vi "Kinesis_XY-AndreTec-Kelly.vi"() -> ()   [LabVIEW 2014]
panel:
  out "Progresso 2":i32=5
  out "Y 4":sgl=0.9991
  out "X 4":sgl=1.0
  out "Y 3":sgl=0.8991
  out "X 3":sgl=0.0001 format="%#_4g"
  out "Tempo de 1 linha 2":u32=9994
  out "Y 2":sgl=0.9991
  out "Y 1":sgl=0.8991
  out "Tempo de 1 linha":u32=10015
  out "X 2":sgl
  out "X 1":sgl=0.999 format="%#_4g"
  in  "Cronometro":bool
  out "millisecond":sgl=332.872
  in  "Aceleração":dbl=1.0
  in  "d (mm)":sgl=0.1
  in  "L (mm)":sgl=1.0
  in  "Iniciar":bool
  out "Progresso":i32=5
  in  "Numero deCiclos":i32=5
  in  "Velocidade":sgl=0.05
  out "Motor Y\nLigado":bool=TRUE
  out "Motor X \nLigado":bool=TRUE
  # "(mm/s)"
  # "(mm/s.s)"
  # "FOCO"
  # "Não Mover"
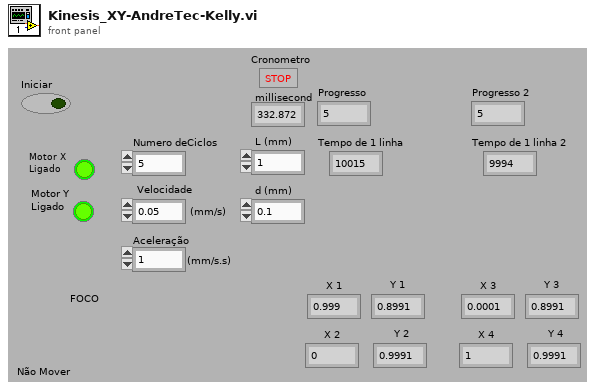
[diagram p1: front panel]
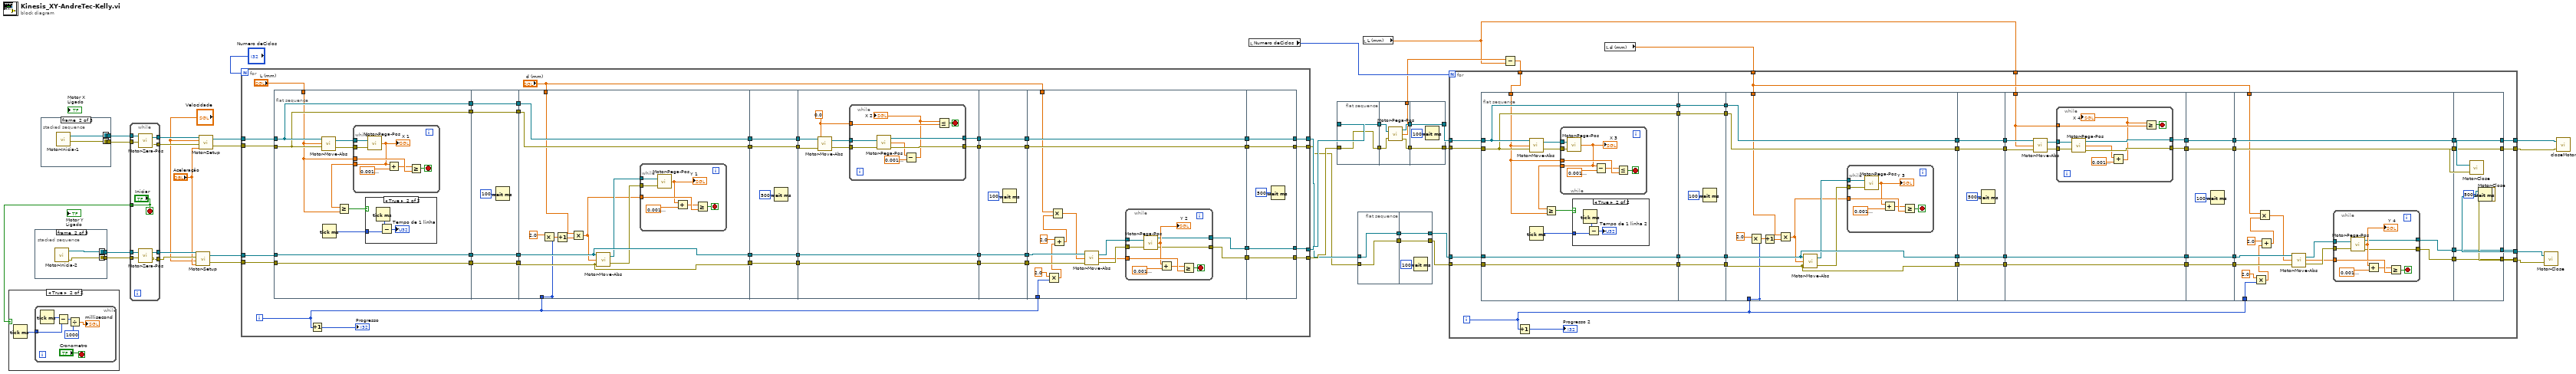
[diagram p0: block diagram]
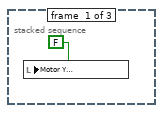
[diagram p5: hidden frame]
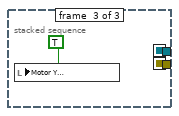
[diagram p6: hidden frame]
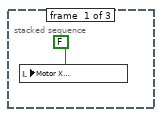
[diagram p7: hidden frame]
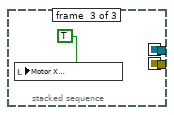
[diagram p8: hidden frame]
diagram:
  n1 = stacked-sequence {
    seq-local: [_ w42 _] -> [_ _ w45]
    seq-local: [_ w41 _] -> [_ _ w44]
    tunnel: [_ _ w45] -> w37
    tunnel: [_ _ w44] -> w36
    frame #0 {
      n2 = local write "Motor Y\nLigado"(FALSE ("Motor3\nLigado")) -> ()
    }
    frame #1 {
      n3 = call "Motor-Inicia-2.vi"() -> ("MG17Motor 2"=w42:refnum<k7>, "error out"=w41:errorcluster)  [unwired: 2 in]
    }
    frame #2 {
      n4 = local write "Motor Y\nLigado"(TRUE ("Motor3\nLigado")) -> ()
    }
  }
  n5 = stacked-sequence {
    seq-local: [_ w48 _] -> [_ _ w51]
    seq-local: [_ w47 _] -> [_ _ w50]
    tunnel: [_ _ w51] -> w39
    tunnel: [_ _ w50] -> w38
    frame #0 {
      n6 = local write "Motor X \nLigado"(FALSE ("x = y?")) -> ()
    }
    frame #1 {
      n7 = call "Motor-Inicia-1.vi"() -> ("MG17Motor 2"=w48:refnum<k7>, "error out"=w47:errorcluster)  [unwired: 1 in]
    }
    frame #2 {
      n8 = local write "Motor X \nLigado"(TRUE ("x = y?")) -> ()
    }
  }
  n9 = while {
    tunnel: w39 -> [w60]
    tunnel: w38 -> [w59]
    tunnel: w37 -> [w58]
    tunnel: w36 -> [w57]
    tunnel: [w56] -> w35
    tunnel: [w55] -> w34
    tunnel: [w54] -> w33
    tunnel: [w53] -> w32
    tunnel: ["Iniciar"] -> w24
    stop <- "Iniciar" stop-if-true
    n10 = call "Motor-Zera-Pos.vi"("error"=w59, "MG17Motor A"=w60) -> ("error out"=w55:errorcluster, "MG17Motor out"=w56:refnum<k7>)
    n11 = call "Motor-Zera-Pos.vi"("error"=w57, "MG17Motor A"=w58) -> ("error out"=w53:errorcluster, "MG17Motor out"=w54:refnum<k7>)
  }
  n12 = case shown="True" w24 {
    frame False {
    }
    frame True {
      n13 = Tick Count (ms)() -> (millisecond timer value=w61:u32)
      n14 = while {
        tunnel: w61 -> [w65]
        stop <- "Cronometro" stop-if-true
        n15 = Tick Count (ms)() -> (millisecond timer value=w67:u32)
        n16 = Subtract(x=w67, y=w65) -> (x-y=w64:u32)
        n17 = Divide(x=w64, y=u32 1000) -> (x/y=→"millisecond":dbl)
      }
    }
  }
  n18 = call "Motor-Setup.vi"("Acc"="Aceleração", "Velocidade"="Velocidade", "error"=w32, "MG17Motor A"=w33) -> ("error out"=w28:errorcluster, "MG17Motor out"=w29:refnum<k7>)
  n19 = call "Motor-Setup.vi"("Acc"="Aceleração", "Velocidade"="Velocidade", "error"=w34, "MG17Motor A"=w35) -> ("error out"=w30:errorcluster, "MG17Motor out"=w31:refnum<k7>)
  n20 = for {
    N: "Numero deCiclos" -> [_]
    tunnel: w31 -> [w107]
    tunnel: w30 -> [w106]
    tunnel: w29 -> [w105]
    tunnel: w28 -> [w104]
    tunnel: [w103] -> w17
    tunnel: [w102] -> w15
    tunnel: [w101] -> w21
    tunnel: [w100] -> w20
    i -> [w70]
    n21 = flat-sequence {
      tunnel: w107 -> [w117]
      tunnel: [w117] -> w99
      tunnel: w106 -> [w116]
      tunnel: [w116] -> w98
      tunnel: w105 -> [w110]
      tunnel: [w110] -> w97
      tunnel: w104 -> [w109]
      tunnel: [w109] -> w96
      tunnel: "L (mm)" -> [w108]
      tunnel: w99 -> [w131]
      tunnel: [w131] -> w95
      tunnel: w98 -> [w130]
      tunnel: [w130] -> w94
      tunnel: w97 -> [w129]
      tunnel: [w129] -> w93
      tunnel: w96 -> [w128]
      tunnel: [w128] -> w92
      tunnel: w95 -> [w140]
      tunnel: [w140] -> w91
      tunnel: w94 -> [w139]
      tunnel: [w139] -> w90
      tunnel: w93 -> [w144]
      tunnel: [w144] -> w89
      tunnel: w92 -> [w143]
      tunnel: [w143] -> w88
      tunnel: "d (mm)" -> [w138]
      tunnel: [w136] -> _
      tunnel: w70 -> [w136]
      tunnel: w91 -> [w155]
      tunnel: [w155] -> w87
      tunnel: w90 -> [w154]
      tunnel: [w154] -> w86
      tunnel: w89 -> [w153]
      tunnel: [w153] -> w85
      tunnel: w88 -> [w152]
      tunnel: [w152] -> w84
      tunnel: w87 -> [w165]
      tunnel: w86 -> [w164]
      tunnel: w85 -> [w158]
      tunnel: [w158] -> w83
      tunnel: w84 -> [w157]
      tunnel: [w157] -> w82
      tunnel: [w160] -> w81
      tunnel: [w159] -> w80
      tunnel: w83 -> [w178]
      tunnel: [w178] -> w79
      tunnel: w82 -> [w177]
      tunnel: [w177] -> w78
      tunnel: w81 -> [w176]
      tunnel: [w176] -> w77
      tunnel: w80 -> [w175]
      tunnel: [w175] -> w76
      tunnel: w79 -> [w194]
      tunnel: w78 -> [w193]
      tunnel: w77 -> [w188]
      tunnel: [w188] -> w75
      tunnel: w76 -> [w187]
      tunnel: [w187] -> w74
      tunnel: [w189] -> w73
      tunnel: [w190] -> w72
      tunnel: w70 -> [w184]
      tunnel: "d (mm)" -> [w186]
      tunnel: [w207] -> w103
      tunnel: w75 -> [w207]
      tunnel: [w206] -> w102
      tunnel: w74 -> [w206]
      tunnel: [w205] -> w101
      tunnel: w73 -> [w205]
      tunnel: [w204] -> w100
      tunnel: w72 -> [w204]
      frame #0 {
        n22 = call "Motor-Move-Abs.vi"("error"=w116, "Posição"=w108, "MG17Motor A"=w117) -> ("error out"=w114:errorcluster, "MG17Motor out"=w115:refnum<k7>)
        n23 = Tick Count (ms)() -> (millisecond timer value=w112:u32)
        n24 = while {
          tunnel: w115 -> [w127]
          tunnel: w114 -> [w126]
          tunnel: w108 -> [w124]
          tunnel: [w123] -> w111
          stop <- w125 stop-if-true
          n25 = call "Motor-Pega-Pos.vi"("MG17Motor 2"=w127, "error out"=w126) -> ("pfPosition"=w123:sgl)  [unwired: 2 out]
          "X 1" <- w123
          n26 = Add(x=w123, y=sgl 0.001) -> (x+y=w121:sgl)
          n27 = Greater Or Equal?(x=w121, y=w124) -> (x >= y?=w125:bool)
        }
        n28 = Greater Or Equal?(x=w111, y=w108) -> (x >= y?=w113:bool)
        n29 = case shown="True" w113 {
          tunnel: w112 -> [_ w119]
          frame False {
          }
          frame True {
            n30 = Tick Count (ms)() -> (millisecond timer value=w120:u32)
            n31 = Subtract(x=w120, y=w119) -> (x-y=→"Tempo de 1 linha":u32)
          }
        }
      }
      frame #1 {
        n32 = Wait (ms)(milliseconds to wait=u32 100) -> ()  [unwired: 1 out]
      }
      frame #2 {
        n33 = Multiply(x=2.0, y=w136) -> (x*y=w135:dbl)
        n34 = Increment(x=w135) -> (x+1=w134:dbl)
        n35 = Multiply(x=w138, y=w134) -> (x*y=w133:dbl)
        n36 = call "Motor-Move-Abs.vi"("error"=w143, "Posição"=w133, "MG17Motor A"=w144) -> ("error out"=w141:errorcluster, "MG17Motor out"=w142:refnum<k7>)
        n37 = while {
          tunnel: w142 -> [w151]
          tunnel: w141 -> [w150]
          tunnel: w133 -> [w148]
          stop <- w149 stop-if-true
          n38 = call "Motor-Pega-Pos.vi"("MG17Motor 2"=w151, "error out"=w150) -> ("pfPosition"=w145:sgl)  [unwired: 2 out]
          "Y 1" <- w145
          n39 = Add(x=w145, y=sgl 0.001) -> (x+y=w146:sgl)
          n40 = Greater Or Equal?(x=w146, y=w148) -> (x >= y?=w149:bool)
        }
      }
      frame #3 {
        n41 = Wait (ms)(milliseconds to wait=u32 500) -> ()  [unwired: 1 out]
      }
      frame #4 {
        w161 = sgl 0.0 ("Posição")
        n42 = call "Motor-Move-Abs.vi"("error"=w164, "Posição"=w161, "MG17Motor A"=w165) -> ("error out"=w162:errorcluster, "MG17Motor out"=w163:refnum<k7>)
        n43 = while {
          tunnel: w163 -> [w174]
          tunnel: w162 -> [w173]
          tunnel: w161 -> [w171]
          tunnel: [w170] -> w160
          tunnel: [w169] -> w159
          stop <- w172 stop-if-true
          n44 = call "Motor-Pega-Pos.vi"("MG17Motor 2"=w174, "error out"=w173) -> ("MG17Motor 3"=w170:refnum<k7>, "pfPosition"=w168:sgl, "error out 2"=w169:errorcluster)
          n45 = Subtract(x=w168, y=sgl 0.001) -> (x-y=w166:sgl)
          "X 2" <- w166
          n46 = Less Or Equal?(x=w166, y=w171) -> (x <= y?=w172:bool)
        }
      }
      frame #5 {
        n47 = Wait (ms)(milliseconds to wait=u32 100) -> ()  [unwired: 1 out]
      }
      frame #6 {
        n48 = Multiply(x=2.0, y=w184) -> (x*y=w182:dbl)
        n49 = Add(x=2.0, y=w182) -> (x+y=w181:dbl)
        n50 = Multiply(x=w186, y=w181) -> (x*y=w180:dbl)
        n51 = call "Motor-Move-Abs.vi"("error"=w193, "Posição"=w180, "MG17Motor A"=w194) -> ("error out"=w191:errorcluster, "MG17Motor out"=w192:refnum<k7>)
        n52 = while {
          tunnel: w192 -> [w203]
          tunnel: w191 -> [w202]
          tunnel: w180 -> [w200]
          tunnel: [w196] -> w189
          tunnel: [w195] -> w190
          stop <- w201 stop-if-true
          n53 = call "Motor-Pega-Pos.vi"("MG17Motor 2"=w203, "error out"=w202) -> ("MG17Motor 3"=w196:refnum<k7>, "pfPosition"=w197:sgl, "error out 2"=w195:errorcluster)
          "Y 2" <- w197
          n54 = Add(x=w197, y=sgl 0.001) -> (x+y=w198:sgl)
          n55 = Greater Or Equal?(x=w198, y=w200) -> (x >= y?=w201:bool)
        }
      }
      frame #7 {
        n56 = Wait (ms)(milliseconds to wait=u32 500 ("millisecond timer value")) -> ()  [unwired: 1 out]
      }
    }
    n57 = Increment(x=w70) -> (x+1=→"Progresso":i32)
  }
  n58 = local read "Numero deCiclos"() -> (w23:i32)
  n59 = flat-sequence {
    tunnel: w21 -> [w210]
    tunnel: w20 -> [w209]
    tunnel: [w209] -> w8
    tunnel: [w210] -> w2
    tunnel: [w214] -> w9
    tunnel: w8 -> [w213]
    tunnel: [w212] -> w7
    tunnel: [w211] -> w6
    tunnel: w2 -> [w215]
    tunnel: [w217] -> w18
    tunnel: [w218] -> w19
    tunnel: w9 -> [w218]
    tunnel: w7 -> [w217]
    frame #0 {
    }
    frame #1 {
      n60 = call "Motor-Pega-Pos.vi"("MG17Motor 2"=w215, "error out"=w213) -> ("MG17Motor 3"=w214:refnum<k7>, "pfPosition"=w211:sgl, "error out 2"=w212:errorcluster)
    }
    frame #2 {
      n61 = Wait (ms)(milliseconds to wait=u32 100) -> ()  [unwired: 1 out]
    }
  }
  n62 = flat-sequence {
    tunnel: w17 -> [w220]
    tunnel: w15 -> [w219]
    tunnel: [w220] -> w4
    tunnel: [w219] -> w3
    tunnel: [w222] -> w14
    tunnel: [w223] -> w16
    tunnel: w4 -> [w223]
    tunnel: w3 -> [w222]
    frame #0 {
    }
    frame #1 {
      n63 = Wait (ms)(milliseconds to wait=u32 100) -> ()  [unwired: 1 out]
    }
  }
  n64 = local read "L (mm)"() -> (w1:sgl)
  n65 = Subtract(x=w6, y=w1) -> (x-y=w5:sgl)
  n66 = local read "d (mm)"() -> (w22:sgl)
  n67 = for {
    N: w23 -> [_]
    tunnel: w19 -> [w264]
    tunnel: w18 -> [w263]
    tunnel: w16 -> [w262]
    tunnel: w14 -> [w261]
    tunnel: [w260] -> w13
    tunnel: [w259] -> w12
    tunnel: [w258] -> w11
    tunnel: [w257] -> w10
    tunnel: w5 -> [w225]
    tunnel: w22 -> [w226]
    tunnel: w1 -> [w224]
    i -> [w228]
    n68 = flat-sequence {
      tunnel: w264 -> [w274]
      tunnel: [w274] -> w256
      tunnel: w263 -> [w273]
      tunnel: [w273] -> w255
      tunnel: w262 -> [w267]
      tunnel: [w267] -> w254
      tunnel: w261 -> [w266]
      tunnel: [w266] -> w253
      tunnel: w225 -> [w265]
      tunnel: w256 -> [w288]
      tunnel: [w288] -> w252
      tunnel: w255 -> [w287]
      tunnel: [w287] -> w251
      tunnel: w254 -> [w286]
      tunnel: [w286] -> w250
      tunnel: w253 -> [w285]
      tunnel: [w285] -> w249
      tunnel: w252 -> [w297]
      tunnel: [w297] -> w248
      tunnel: w251 -> [w296]
      tunnel: [w296] -> w247
      tunnel: w250 -> [w301]
      tunnel: [w301] -> w246
      tunnel: w249 -> [w300]
      tunnel: [w300] -> w245
      tunnel: w226 -> [w295]
      tunnel: [w293] -> _
      tunnel: w228 -> [w293]
      tunnel: w248 -> [w312]
      tunnel: [w312] -> w244
      tunnel: w247 -> [w311]
      tunnel: [w311] -> w243
      tunnel: w246 -> [w310]
      tunnel: [w310] -> w242
      tunnel: w245 -> [w309]
      tunnel: [w309] -> w241
      tunnel: w244 -> [w322]
      tunnel: w243 -> [w321]
      tunnel: w242 -> [w316]
      tunnel: [w316] -> w240
      tunnel: w241 -> [w315]
      tunnel: [w315] -> w239
      tunnel: [w318] -> w238
      tunnel: [w317] -> w237
      tunnel: w224 -> [w314]
      tunnel: w240 -> [w335]
      tunnel: [w335] -> w236
      tunnel: w239 -> [w334]
      tunnel: [w334] -> w235
      tunnel: w238 -> [w333]
      tunnel: [w333] -> w234
      tunnel: w237 -> [w332]
      tunnel: [w332] -> w233
      tunnel: w236 -> [w351]
      tunnel: w235 -> [w350]
      tunnel: w234 -> [w345]
      tunnel: [w345] -> w232
      tunnel: w233 -> [w344]
      tunnel: [w344] -> w231
      tunnel: [w346] -> w230
      tunnel: [w347] -> w229
      tunnel: w228 -> [w341]
      tunnel: w226 -> [w343]
      tunnel: [w364] -> w260
      tunnel: w232 -> [w364]
      tunnel: [w363] -> w259
      tunnel: w231 -> [w363]
      tunnel: [w362] -> w258
      tunnel: w230 -> [w362]
      tunnel: [w361] -> w257
      tunnel: w229 -> [w361]
      frame #0 {
        n69 = call "Motor-Move-Abs.vi"("error"=w273, "Posição"=w265, "MG17Motor A"=w274) -> ("error out"=w271:errorcluster, "MG17Motor out"=w272:refnum<k7>)
        n70 = Tick Count (ms)() -> (millisecond timer value=w269:u32)
        n71 = while {
          tunnel: w272 -> [w284]
          tunnel: w271 -> [w283]
          tunnel: w265 -> [w281]
          tunnel: [w278] -> w268
          stop <- w282 stop-if-true
          n72 = call "Motor-Pega-Pos.vi"("MG17Motor 2"=w284, "error out"=w283) -> ("pfPosition"=w278:sgl)  [unwired: 2 out]
          "X 3" <- w278
          n73 = Subtract(x=w278, y=sgl 0.001) -> (x-y=w279:sgl)
          n74 = Less Or Equal?(x=w279, y=w281) -> (x <= y?=w282:bool)
        }
        n75 = Greater Or Equal?(x=w268, y=w265) -> (x >= y?=w270:bool)
        n76 = case shown="True" w270 {
          tunnel: w269 -> [_ w276]
          frame False {
          }
          frame True {
            n77 = Tick Count (ms)() -> (millisecond timer value=w277:u32)
            n78 = Subtract(x=w277, y=w276) -> (x-y=→"Tempo de 1 linha 2":u32)
          }
        }
      }
      frame #1 {
        n79 = Wait (ms)(milliseconds to wait=u32 100) -> ()  [unwired: 1 out]
      }
      frame #2 {
        n80 = Multiply(x=2.0, y=w293) -> (x*y=w292:dbl)
        n81 = Increment(x=w292) -> (x+1=w291:dbl)
        n82 = Multiply(x=w295, y=w291) -> (x*y=w290:dbl)
        n83 = call "Motor-Move-Abs.vi"("error"=w300, "Posição"=w290, "MG17Motor A"=w301) -> ("error out"=w298:errorcluster, "MG17Motor out"=w299:refnum<k7>)
        n84 = while {
          tunnel: w299 -> [w308]
          tunnel: w298 -> [w307]
          tunnel: w290 -> [w305]
          stop <- w306 stop-if-true
          n85 = call "Motor-Pega-Pos.vi"("MG17Motor 2"=w308, "error out"=w307) -> ("pfPosition"=w302:sgl)  [unwired: 2 out]
          "Y 3" <- w302
          n86 = Add(x=w302, y=sgl 0.001) -> (x+y=w303:sgl)
          n87 = Greater Or Equal?(x=w303, y=w305) -> (x >= y?=w306:bool)
        }
      }
      frame #3 {
        n88 = Wait (ms)(milliseconds to wait=u32 500) -> ()  [unwired: 1 out]
      }
      frame #4 {
        n89 = call "Motor-Move-Abs.vi"("error"=w321, "Posição"=w314, "MG17Motor A"=w322) -> ("error out"=w319:errorcluster, "MG17Motor out"=w320:refnum<k7>)
        n90 = while {
          tunnel: w320 -> [w331]
          tunnel: w319 -> [w330]
          tunnel: w314 -> [w328]
          tunnel: [w327] -> w318
          tunnel: [w326] -> w317
          stop <- w329 stop-if-true
          n91 = call "Motor-Pega-Pos.vi"("MG17Motor 2"=w331, "error out"=w330) -> ("MG17Motor 3"=w327:refnum<k7>, "pfPosition"=w323:sgl, "error out 2"=w326:errorcluster)
          n92 = Add(x=w323, y=sgl 0.001) -> (x+y=w324:sgl)
          "X 4" <- w324
          n93 = Greater Or Equal?(x=w324, y=w328) -> (x >= y?=w329:bool)
        }
      }
      frame #5 {
        n94 = Wait (ms)(milliseconds to wait=u32 100) -> ()  [unwired: 1 out]
      }
      frame #6 {
        n95 = Multiply(x=2.0, y=w341) -> (x*y=w339:dbl)
        n96 = Add(x=2.0, y=w339) -> (x+y=w338:dbl)
        n97 = Multiply(x=w343, y=w338) -> (x*y=w337:dbl)
        n98 = call "Motor-Move-Abs.vi"("error"=w350, "Posição"=w337, "MG17Motor A"=w351) -> ("error out"=w348:errorcluster, "MG17Motor out"=w349:refnum<k7>)
        n99 = while {
          tunnel: w349 -> [w360]
          tunnel: w348 -> [w359]
          tunnel: w337 -> [w357]
          tunnel: [w353] -> w346
          tunnel: [w352] -> w347
          stop <- w358 stop-if-true
          n100 = call "Motor-Pega-Pos.vi"("MG17Motor 2"=w360, "error out"=w359) -> ("MG17Motor 3"=w353:refnum<k7>, "pfPosition"=w354:sgl, "error out 2"=w352:errorcluster)
          "Y 4" <- w354
          n101 = Add(x=w354, y=sgl 0.001) -> (x+y=w355:sgl)
          n102 = Greater Or Equal?(x=w355, y=w357) -> (x >= y?=w358:bool)
        }
      }
      frame #7 {
        n103 = Wait (ms)(milliseconds to wait=u32 500 ("millisecond timer value")) -> ()  [unwired: 1 out]
      }
    }
    n104 = Increment(x=w228) -> (x+1=→"Progresso 2":i32)
  }
  n105 = call "Motor-Close.vi"("error out"=w12, "MG17Motor 3"=w13) -> ()  [unwired: 1 in]
  n106 = call "Motor-Close.vi"("error out"=w10, "MG17Motor 3"=w11) -> ()  [unwired: 1 in]
  n107 = call "Motor-Close.vi"("error out"=w10, "MG17Motor 3"=w11) -> ()  [unwired: 1 in]
  n108 = call "closeMotor.vi"(1:w12, ".NET Refnum in"=w13) -> ()  [unwired: 1 in]
